vi "Exit Event Loop.vi"(8 "error in (no error)":errorcluster, 11 "GUI Container in":refnum<class "GUI Container.lvclass">) -> (0 "error out":errorcluster, 3 "GUI Container out":refnum<class "GUI Container.lvclass">)   [LabVIEW 2023, in "GUI Views.lvlib" / "GUI Container.lvclass"]
doc: "This method must be called in the \"Actor Core.vi\" of the subclass of the GUI Container. If in this \"Actor Core.vi\" the method \"Register to Container Events.vi\" was called and the helper event loop is listening to the corresponding event calling this method will cause the helper event loop to exit. This is useful to allow the exit of the helper loop when the stop message of the actor is received. Calling this method is optional. See the examples for an illustration of its usage."
uses:
  GUI Container.lvclass
  GUI Container.lvclass/GUI Container.ctl
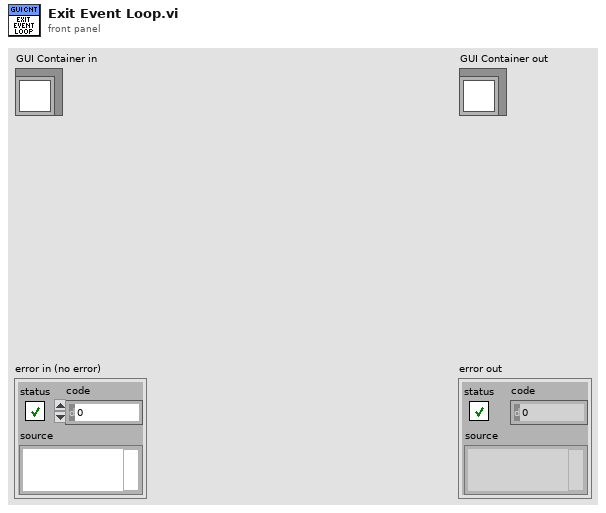
[diagram p1: front panel]
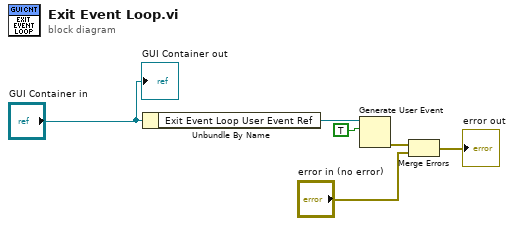
[diagram p0: block diagram]
diagram:
  n1 = Unbundle By Name("GUI Container in") -> ("Exit Event Loop User Event Ref"=w4:refnum<user-event>)
  n2 = Generate User Event(user event=w4, event data cluster=TRUE ("event data")) -> (error out=w1:errorcluster)  [unwired: 2 in, 1 out]
  n3 = Merge Errors(w1, "error in (no error)") -> (→"error out":errorcluster)
  "GUI Container out" <- "GUI Container in"
